vi "Query Alarm Status.vi"(8 "error in (no error)":errorcluster, 11 "GEN40-38-LAN in":refnum<class "GEN40-38-LAN.lvclass">) -> (0 "error out":errorcluster, 2 "Alarm":bool, 3 "GEN40-38-LAN out":refnum<class "GEN40-38-LAN.lvclass">)   [LabVIEW 2018, in "GEN40-38-LAN.lvlib" / "GEN40-38-LAN.lvclass"]
uses:
  GEN40-38-LAN.lvclass
  PPLs/Power Supply/Parent/Power_Supply.lvlibp/Power Supply.lvclass
  C:/Projects/LabVIEW/PPLs/Power Supply/Parent/Power_Supply.lvlibp/Power Supply.lvclass
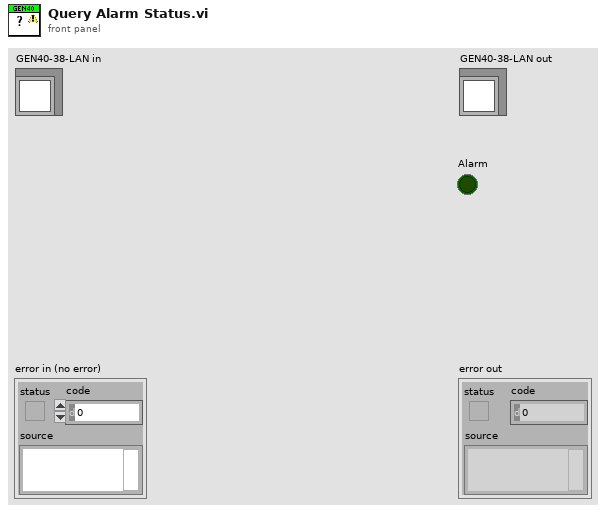
[diagram p1: front panel]
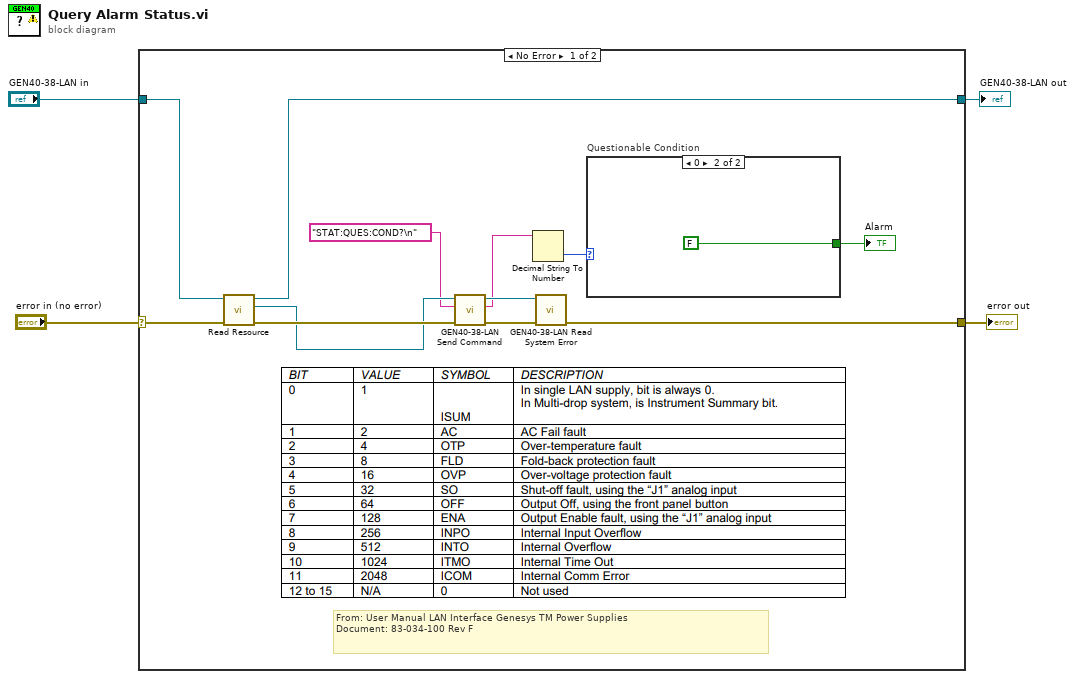
[diagram p0: block diagram]
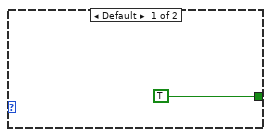
[diagram p2: hidden frame]
diagram:
  n1 = case shown="No Error" "error in (no error)" {
    selector: "error in (no error)" -> [w16 w20]
    tunnel: [w9 w20] -> w3
    tunnel: [w14 w19] -> w2
    tunnel: "GEN40-38-LAN in" -> [w15 w19]
    frame No Error {
      # "From: User Manual LAN Interface Genesys TM Power Supplies\nDocument: 83-034-100 Rev F"
      n2 = call "Read Resource.vi"("error in"=w16, "Power Supply in"=w15) -> ("error out"=w13:errorcluster, "Resource"=w12:refnum<visa-resource-name>, "Power Supply out"=w14:refnum<class "GEN40-38-LAN.lvclass">)  [unwired: 7 in]
      n3 = call "GEN40-38-LAN Send Command.vi"("error in (no error)"=w13, "Command"="STAT:QUES:COND?\n", "VISA resource name"=w12) -> ("error out"=w10:errorcluster, "Response"=w7:string, "VISA resource name out"=w11:refnum<visa-resource-name>)  [unwired: 6 in]
      n4 = Decimal String To Number(string=w7) -> (number=w6:i32)  [unwired: 2 in, 1 out]
      n5 = call "GEN40-38-LAN Read System Error.vi"("error in (no error)"=w10, "Resource"=w11) -> ("error out"=w9:errorcluster)  [unwired: 9 in]
      n6 = case "Questionable Condition" shown="0" w6 {
        tunnel: [TRUE FALSE] -> w5
        frame Default {
          # "From table below, these values are considered an Alarm status"
        }
        frame 0 {
          # "From table below, these values are not considered an Alarm status"
        }
      }
      "Alarm" <- w5
    }
    frame Error {
    }
  }
  "error out" <- w3
  "GEN40-38-LAN out" <- w2
